vi "from string 1.0.vi"(8 "error in (no error)":errorcluster, 10 "data":string, 11 "Benchmark PID configuration in":refnum<class "Benchmark PID configuration.lvclass">) -> (0 "error out":errorcluster, 3 "Benchmark PID configuration out":refnum<class "Benchmark PID configuration.lvclass">)   [LabVIEW 2018, in "Benchmark PID configuration.lvclass"]
uses:
  Benchmark PID configuration.lvclass
  <vilib>/NI/Tag Bus Module Framework/channel/TBM channel.lvclass
  Line.ctl
  Benchmark PID configuration.lvclass/Benchmark PID configuration.ctl
  <vilib>/NI/Configuration Framework/serializable configuration/NISE_CEF_serializable configuration.lvclass
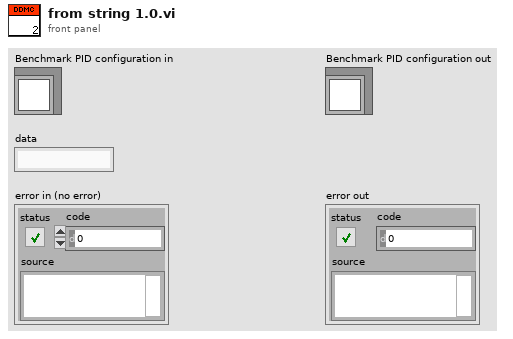
[diagram p1: front panel]
types:
  T1 = typedef "Benchmark PID configuration.lvclass/Line.ctl" = cluster{"PID Name":string, "Setpoint":refnum<class "TBM channel.lvclass">, "Variable":refnum<class "TBM channel.lvclass">, "Output":refnum<class "TBM channel.lvclass">}
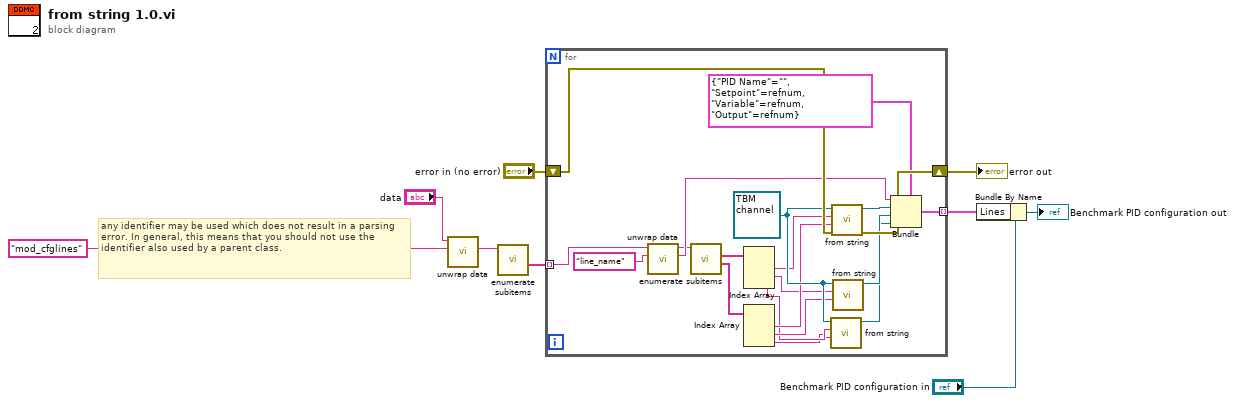
[diagram p0: block diagram]
diagram:
  # "any identifier may be used which does not result in a parsing error. In general, this means that you should not use the identifier also used by a parent class."
  n1 = call <vilib>:"unwrap data.vi"("identifier"="mod_cfglines", "data to unwrap"="data") -> ("unwrapped data"=w7:string)  [unwired: 8 in, 1 out]
  n2 = call <vilib>:"enumerate subitems.vi"("data to enumerate"=w7) -> ("associated data"=w1:string[])  [unwired: 8 in, 2 out]
  n3 = for {
    shift-right: [w29] -> w9
    shift-left: "error in (no error)" -> [w28]
    tunnel: [w26] -> w8 mode=indexing
    tunnel: w1 -> [w20] mode=indexing
    w22 = refnum<class "TBM channel.lvclass"> refnum ("channel in")
    n4 = call <vilib>:"unwrap data.vi"("identifier"="line_name", "data to unwrap"=w20) -> ("unwrapped data"=w19:string, "remaining string"=w18:string)  [unwired: 8 in]
    n5 = call <vilib>:"enumerate subitems.vi"("data to enumerate"=w18) -> ("associated data"=w16:string[], "discovered subitems"=w17:string[])  [unwired: 8 in, 1 out]
    n6 = Index Array(array=w17) -> (element #1=w15:string, element #2=w13:string, element #3=w11:string)  [unwired: 3 in]
    n7 = Index Array(array=w16) -> (element #1=w14:string, element #2=w12:string, element #3=w10:string)  [unwired: 3 in]
    n8 = call-dynamic "from string.vi"("channel data"=w10, "identifier"=w11, "channel in"=w22) -> ("channel out"=w23:refnum<class "TBM channel.lvclass">)  [unwired: 7 in, 1 out]
    n9 = call-dynamic "from string.vi"("error in"=w28, "channel data"=w14, "identifier"=w15, "channel in"=w22) -> ("error out"=w29:errorcluster, "channel out"=w25:refnum<class "TBM channel.lvclass">)  [unwired: 6 in]
    n10 = call-dynamic "from string.vi"("channel data"=w12, "identifier"=w13, "channel in"=w22) -> ("channel out"=w24:refnum<class "TBM channel.lvclass">)  [unwired: 7 in, 1 out]
    n11 = Bundle(cluster=T1 {"PID Name"="", "Setpoint"=refnum, "Variable"=refnum, "Output"=refnum} ("Line"), "PID Name"=w19, "Setpoint"=w25, "Variable"=w24, "Output"=w23) -> (w26:T1)
  }
  "error out" <- w9
  n12 = Bundle By Name(cluster="Benchmark PID configuration in", "Lines"=w8) -> (→"Benchmark PID configuration out":refnum<class "Benchmark PID configuration.lvclass">)
